vi "LeyboldTurbo_Test.vi"() -> ()   [LabVIEW 2019]
doc: "Example VI to demonstrate the use of the Oerlikon Leybold TMP driver."
uses:
  <instrlib>/Leybold TURBOVAC/Leybold TURBOVAC.lvlib
panel:
  in  "SN":string="240804204"
  out "temp_motor":i32 caption="Motor temp. [°C]"
  out "status_error":u32(colorbox) caption="Status"
  out "control_word":bool[](array[boolean])
  in  "Reset in init":bool
  out "P179":bool
  in  "P179_sp":bool=TRUE
  out "time_meas":timestamp caption="Last update" format="%<%Y-%m-%d %H:%M:%S>T"
  out "status_cont":bool caption="Control status"
  in  "set_P182":bool
  in  "P182_sp":dbl format="%.1f"
  out "P182":dbl format="%.1f"
  in  "freq_nom":u16 caption="Nominal frequency" max=700
  in  "interval":u32=1000
  in  "set_nominal_freq":bool
  in  "standby":bool caption="Standby"
  in  "remote_cont":bool caption="Remote Control"
  in  "operate":bool caption="Operate"
  out "Warnings / Errors":string
  out "Status values":T1
  out "Status word":T2
  in  "stop":bool
  in  "VISA":refnum<visa-resource-name>="COM43"
  # "Leybold TURBOVAC 1350iR + TURBO.DRIVE 500e"
  # "Turbo 1: 240804202\nTurbo 2: 240804204"
  # "ms"
  # "0:  Start/Stop"
  # "sec"
  # "10:  Enable process data"
  # "sec"
  # "Hz"
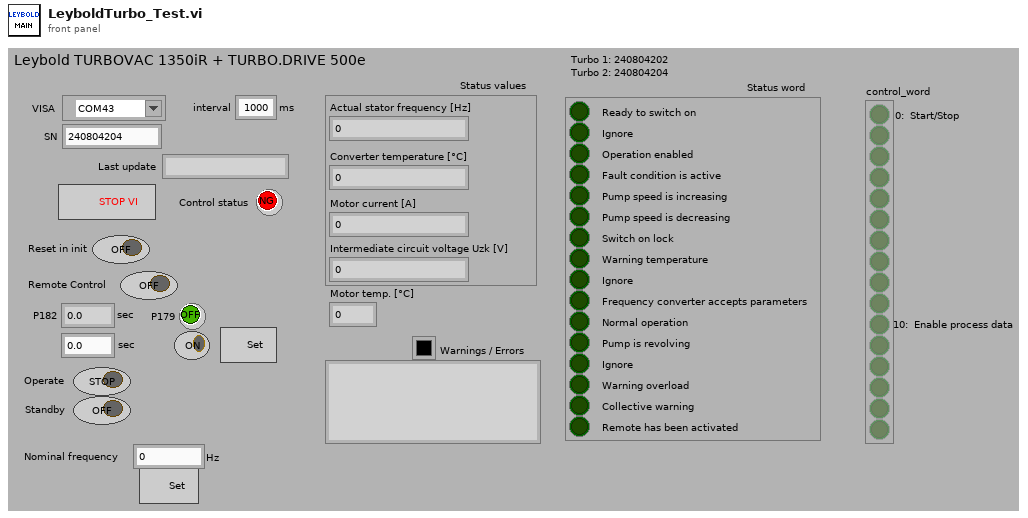
[diagram p1: front panel]
types:
  T1 = cluster{"Actual stator frequency [Hz]":u16, "Converter temperature [°C]":u16, "Motor current [A]":dbl, "Intermediate circuit voltage Uzk [V]":dbl}
  T2 = cluster{"Ready to switch on":bool, "Ignore":bool, "Operation enabled":bool, "Fault condition is active":bool, "Pump speed is increasing":bool, "Pump speed is decreasing":bool, "Switch on lock":bool, "Warning temperature":bool, "Ignore":bool, "Frequency converter accepts parameters":bool, "Normal operation":bool, "Pump is revolving":bool, "Ignore":bool, "Warning overload":bool, "Collective warning":bool, "Remote has been activated":bool}
  T3 = typedef "Leybold TURBOVAC.lvlib/Device Parameters Indicator.ctl" = cluster{"Length of data block":u8, "Converter address":u8, "Converter type":T4, "PZD1":u16, "PZD2":u16}
  T4 = typedef "Leybold TURBOVAC.lvlib/Converter Type Indicator.ctl" = u16
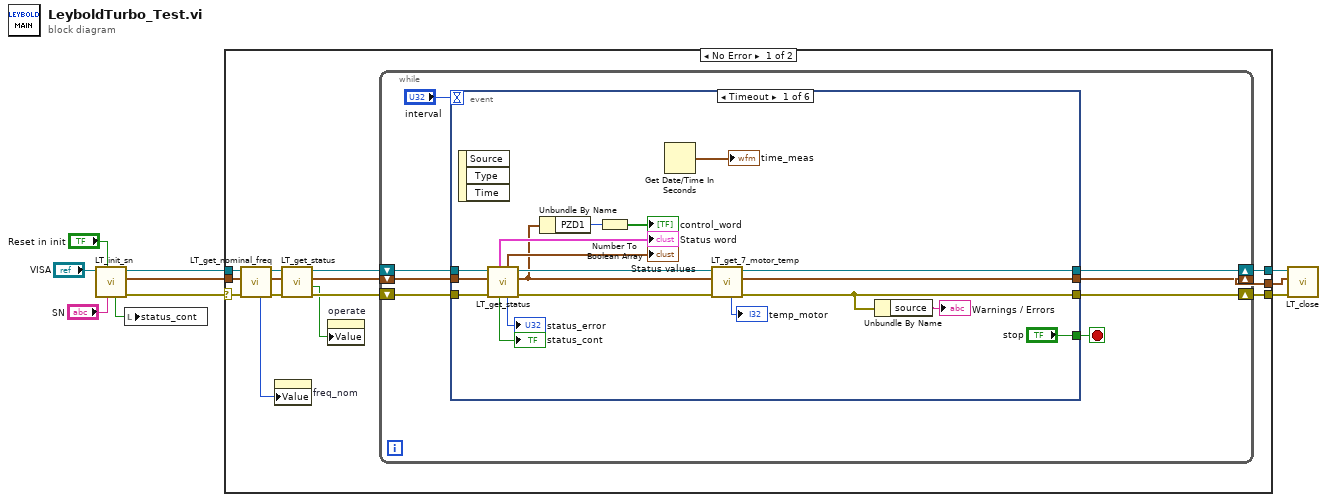
[diagram p0: block diagram]
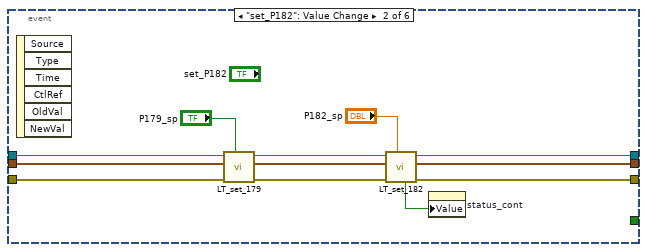
[diagram p2: hidden frame]
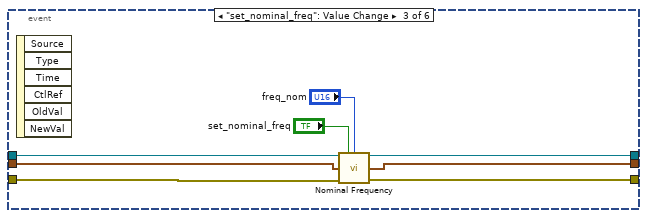
[diagram p3: hidden frame]
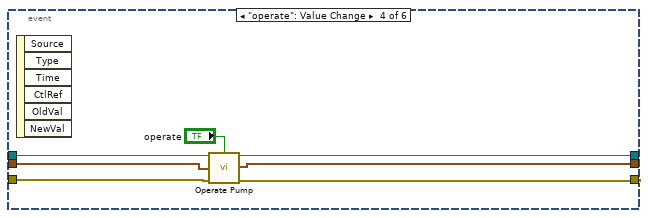
[diagram p4: hidden frame]
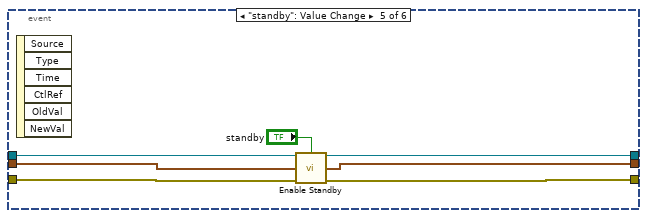
[diagram p5: hidden frame]
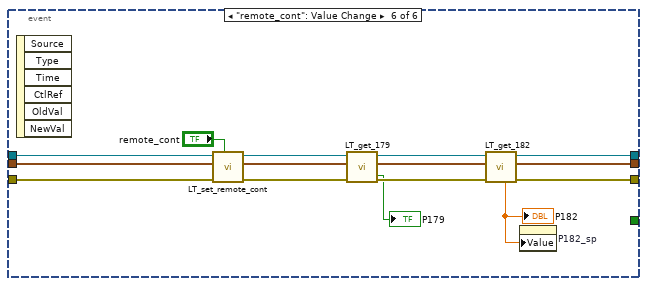
[diagram p6: hidden frame]
diagram:
  n1 = call "LT_init_sn.vi"("SN"="SN", "do_reset"="Reset in init", "VISA in"="VISA") -> ("error out"=w7:errorcluster, "dev_param_out"=w8:T3, "VISA out"=w9:refnum<visa-resource-name>, "status"=w1:bool)  [unwired: 5 in]
  n2 = local write "status_cont"(w1) -> ()
  n3 = case shown="No Error" w7 {
    selector: w7 -> [w19 w101]
    tunnel: w9 -> [w21 w102]
    tunnel: w8 -> [w20 w103]
    tunnel: [w24 w102] -> w6
    tunnel: [w23 w103] -> w4
    tunnel: [w22 w101] -> w5
    frame No Error {
      n4 = call "LT_get_nominal_freq.vi"("error in"=w19, "dev_param_in"=w20, "VISA in"=w21) -> ("error out"=w12:errorcluster, "dev_param_out"=w11:T3, "VISA out"=w13:refnum<visa-resource-name>, "frequency"=w18:i32)  [unwired: 5 in]
      n5 = property on="freq_nom" class="DigNum (strict)"("Value"=w18) -> ()  [unwired: 2 in, 2 out]
      n6 = call "LT_get_status.vi"("error in"=w12, "dev_param_in"=w11, "VISA in"=w13) -> ("error out"=w16:errorcluster, "op_enabled"=w14:bool, "dev_param_out"=w15:T3, "VISA out"=w17:refnum<visa-resource-name>)  [unwired: 1 in, 4 out]
      n7 = property on="operate" class="Bool (strict)"("Value"=w14) -> ()  [unwired: 2 in, 2 out]
      n8 = while {
        shift-right: [w27] -> w23
        shift-left: w15 -> [w28]
        shift-right: [w26] -> w22
        shift-left: w16 -> [w30]
        shift-right: [w31] -> w24
        shift-left: w17 -> [w29]
        stop <- w32 stop-if-true
        n9 = event shown="[0] Timeout" {
          selector: _ -> [_ _ _ _ _ _]
          dyn-events: _ -> [_ _ _ _ _ _]
          timeout: "interval" -> [_ _ _ _ _ _]
          tunnel: ["stop" _ _ _ _ _] -> w32
          tunnel: [w38 w63 w66 w74 w81 w100] -> w31
          tunnel: w30 -> [w47 w54 w67 w75 w82 w91]
          tunnel: w29 -> [w48 w57 w69 w77 w84 w90]
          tunnel: w28 -> [w46 w53 w68 w76 w83 w89]
          tunnel: [w36 w61 w65 w73 w80 w99] -> w27
          tunnel: [w34 w62 w64 w72 w79 w98] -> w26
          event Timeout {
            n10 = event-data() -> ()  [unwired: 1 in, 3 out]
            n11 = call "LT_get_status.vi"("error in"=w47, "dev_param_in"=w46, "VISA in"=w48) -> ("error out"=w35:errorcluster, "dev_param_out"=w37:T3, "VISA out"=w39:refnum<visa-resource-name>, "status_error"=→"status_error":u32, "Status values"=→"Status values":T1, "status_cont"=→"status_cont":bool, "Status word"=→"Status word":T2)  [unwired: 1 in, 1 out]
            n12 = Unbundle By Name(w37) -> ("PZD1"=w42:u16)
            n13 = Number To Boolean Array(number=w42) -> (Boolean array=→"control_word":bool[])
            n14 = Get Date/Time In Seconds() -> (seconds since 1Jan1904=→"time_meas":timestamp)
            n15 = call "LT_get_7_motor_temp.vi"("error in"=w35, "dev_param_in"=w37, "VISA in"=w39) -> ("error out"=w34:errorcluster, "dev_param_out"=w36:T3, "VISA out"=w38:refnum<visa-resource-name>, "temp"=→"temp_motor":i32)  [unwired: 5 in]
            n16 = Unbundle By Name(w34) -> ("source"=→"Warnings / Errors":string)
          }
          event "set_P182": Value Change {
            n17 = event-data() -> ()  [unwired: 1 in, 6 out]
            n18 = call "LT_set_179.vi"("P179"="P179_sp", "error in"=w54, "dev_param_in"=w53, "VISA in"=w57) -> ("error out"=w55:errorcluster, "dev_param_out"=w56:T3, "VISA out"=w58:refnum<visa-resource-name>)  [unwired: 4 in, 1 out]
            n19 = call "LT_set_182.vi"("sec"="P182_sp", "error in"=w55, "dev_param_in"=w56, "VISA in"=w58) -> ("error out"=w62:errorcluster, "dev_param_out"=w61:T3, "VISA out"=w63:refnum<visa-resource-name>, "status"=w59:bool)  [unwired: 4 in]
            n20 = property on="status_cont" class="Bool (strict)"("Value"=w59) -> ()  [unwired: 2 in, 2 out]
          }
          event "set_nominal_freq": Value Change {
            n21 = event-data() -> ()  [unwired: 1 in, 6 out]
            n22 = call <instrlib>:"Nominal Frequency.vi"("VISA resource name"=w69, "Change nominal frequency (F: off)"="set_nominal_freq", "Nominal frequency (1000)"="freq_nom", "Device parameters"=w68, "error in (no error)"=w67) -> ("VISA resource name out"=w66:refnum<visa-resource-name>, "Device parameters out"=w65:T3, "error out"=w64:errorcluster)  [unwired: 8 in]
          }
          event "operate": Value Change {
            n23 = event-data() -> ()  [unwired: 1 in, 6 out]
            n24 = call <instrlib>:"Operate Pump.vi"("VISA resource name"=w77, "Operate pump (F: off)"="operate", "Device parameters"=w76, "error in (no error)"=w75) -> ("VISA resource name out"=w74:refnum<visa-resource-name>, "Device parameters out"=w73:T3, "error out"=w72:errorcluster)  [unwired: 9 in]
          }
          event "standby": Value Change {
            n25 = event-data() -> ()  [unwired: 1 in, 6 out]
            n26 = call <instrlib>:"Enable Standby.vi"("VISA resource name"=w84, "Activate Standy (F: off)"="standby", "Device parameters"=w83, "error in (no error)"=w82) -> ("VISA resource name out"=w81:refnum<visa-resource-name>, "Device parameters out"=w80:T3, "error out"=w79:errorcluster)  [unwired: 9 in]
          }
          event "remote_cont": Value Change {
            n27 = event-data() -> ()  [unwired: 1 in, 6 out]
            n28 = call "LT_set_remote_cont.vi"("remote_cont"="remote_cont", "error in"=w91, "dev_param_in"=w89, "VISA in"=w90) -> ("error out"=w92:errorcluster, "dev_param_out"=w87:T3, "VISA out"=w88:refnum<visa-resource-name>)  [unwired: 4 in, 1 out]
            n29 = call "LT_get_179.vi"("error in"=w92, "dev_param_in"=w87, "VISA in"=w88) -> ("error out"=w95:errorcluster, "dev_param_out"=w94:T3, "VISA out"=w96:refnum<visa-resource-name>, "P179"=→"P179":bool)  [unwired: 5 in]
            n30 = call "LT_get_182.vi"("error in"=w95, "dev_param_in"=w94, "VISA in"=w96) -> ("error out"=w98:errorcluster, "dev_param_out"=w99:T3, "VISA out"=w100:refnum<visa-resource-name>, "sec"=w97:dbl)  [unwired: 5 in]
            "P182" <- w97
            n31 = property on="P182_sp" class="DigNum (strict)"("Value"=w97) -> ()  [unwired: 2 in, 2 out]
          }
        }
      }
    }
    frame Error {
    }
  }
  n32 = call "LT_close.vi"("error in"=w5, "dev_param_in"=w4, "VISA in"=w6) -> ()  [unwired: 9 in]
